vi "Read TDMS File.vi"(8 "error in":errorcluster, 11 "File Path":path) -> (0 "error out":errorcluster, 3 "Data Out":dbl[][](array[numeric]) format="%0.2f")   [LabVIEW 2021]
doc: "Reads data from a .tdms file."
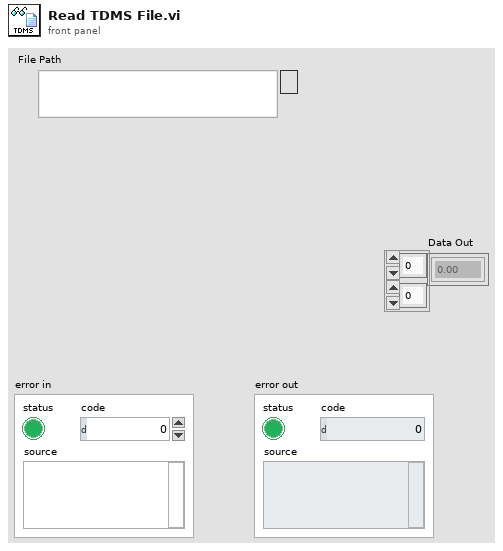
[diagram p1: front panel]
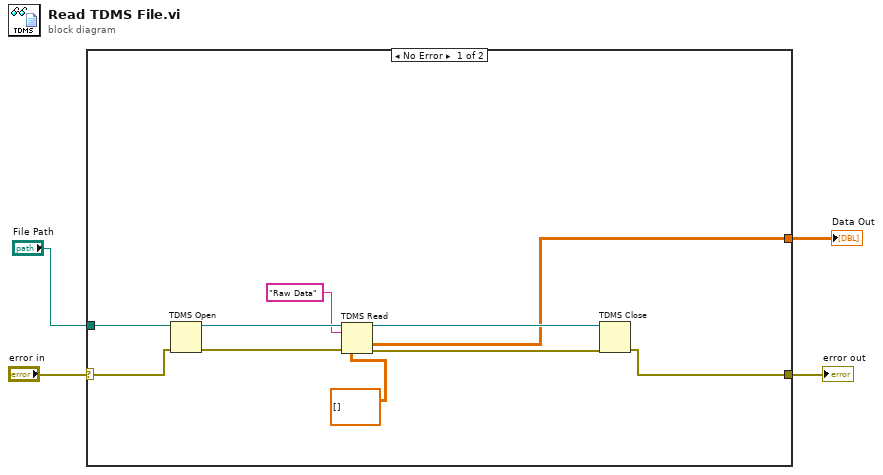
[diagram p0: block diagram]
diagram:
  n1 = case shown="No Error" "error in" {
    selector: "error in" -> [w14 w15]
    tunnel: [w8 w15] -> w3
    tunnel: "File Path" -> [w13 _]
    tunnel: [w5 _] -> w1
    frame No Error {
      n2 = TDMS Open(8:w14, 11:w13) -> (0:w11:errorcluster, 3:w12:refnum<k34>)  [unwired: 5 in]
      n3 = TDMS Read(0:w12, 5:"Raw Data" ("group name in"), 11:w11, 12:dbl[][] [] ("Data")) -> (4:w10:refnum<k34>, 10:w5:dbl[][], 15:w9:errorcluster)  [unwired: 4 in, 3 out]
      n4 = TDMS Close(8:w9, 11:w10) -> (0:w8:errorcluster)  [unwired: 1 out]
    }
    frame Error {
    }
  }
  "error out" <- w3
  "Data Out" <- w1
